vi "Adjust 1D Array to want Size.vi"(10 "y":i32=100, 11 "1D Input":dbl[](array[numeric])) -> (3 "1D Output":dbl[](array[numeric]))   [LabVIEW 2021]
doc: "向HMI写数组时，先在HMI里面配置X和Y的数组大小，OPC里面限制float大小为127，实际使用100.\n当写入的数组不等于100时，HMI上面不显示波形。\n故要调整输入数组的大小。多的去掉，小的补充。\n2015-05-26 09:55:54\n蒋松\njiangsong@outlook.com"
panel:
  out "Waveform Graph":dbl[](graph)
  out "size(s)":i32
  in  "Numeric":i32
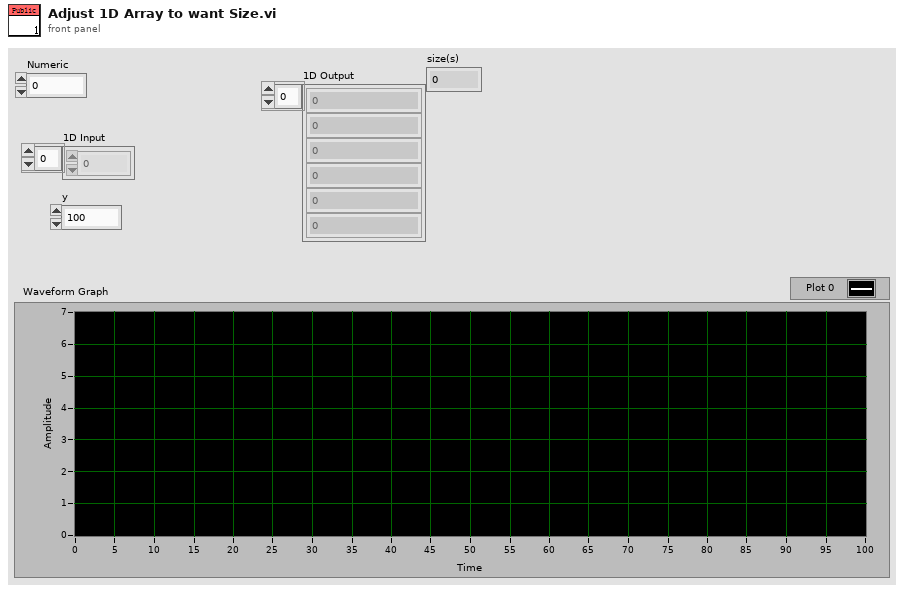
[diagram p1: front panel]
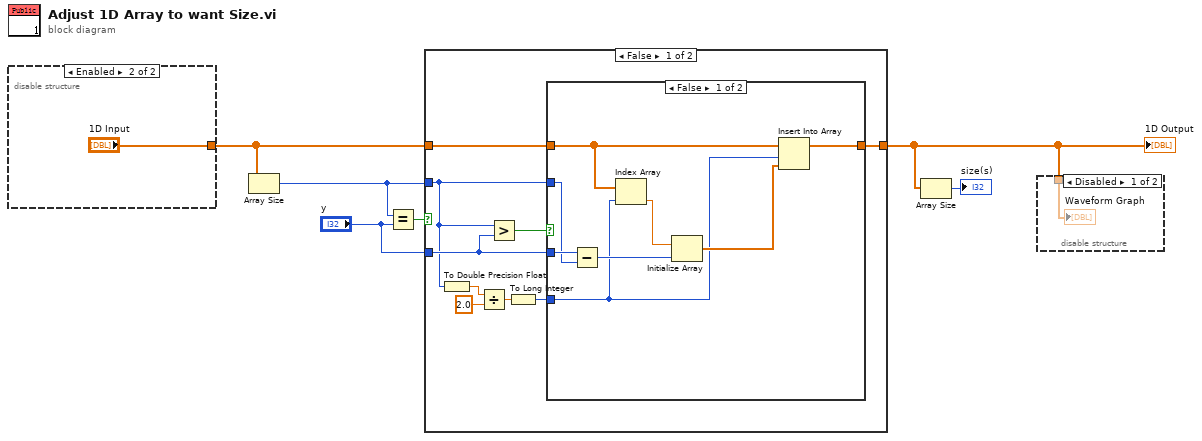
[diagram p0: block diagram]
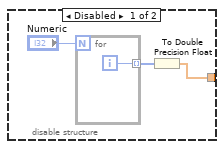
[diagram p3: hidden frame]
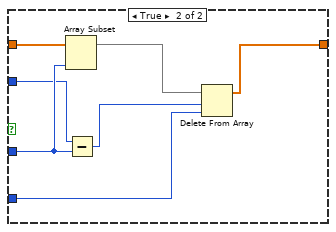
[diagram p4: hidden frame]
diagram:
  n1 = disable-structure shown="Enabled" {
    disable-tunnel: [w7 "1D Input"] -> w3
    frame Disabled {
      n2 = for {
        N: "Numeric" -> [_]
        tunnel: [w10] -> w8 mode=indexing
        i -> [w10]
      }
      n3 = To Double Precision Float(number=w8) -> (double precision float=w7:dbl[])
    }
    frame Enabled {
    }
  }
  n4 = Array Size(array=w3) -> (size(s)=w5:i32)
  n5 = Equal?(x=w5, y="y") -> (x = y?=w6:bool)
  n6 = case shown="False" w6 {
    tunnel: [w18 w36] -> w1
    tunnel: w3 -> [w19 w36]
    tunnel: w5 -> [w13 _]
    tunnel: "y" -> [w17 _]
    frame False {
      n7 = To Double Precision Float(number=w13) -> (double precision float=w15:dbl)
      n8 = Divide(x=w15, y=2.0) -> (x/y=w16:dbl)
      n9 = Greater?(x=w13, y=w17) -> (0:w20:bool)
      n10 = To Long Integer(number=w16) -> (32bit integer=w12:i32)
      n11 = case shown="False" w20 {
        tunnel: w19 -> [w25 w35]
        tunnel: [w23 w30] -> w18
        tunnel: w17 -> [w28 w34]
        tunnel: w13 -> [w22 w32]
        tunnel: w12 -> [w21 w29]
        frame False {
          n12 = Subtract(x=w28, y=w22) -> (x-y=w26:i32)
          n13 = Index Array(array=w25, index=w21) -> (element=w27:dbl)
          n14 = Initialize Array(w27, w26) -> (w24:dbl[])
          n15 = Insert Into Array(array=w25, index=w21, new element=w24) -> (w23:dbl[])
        }
        frame True {
          n16 = Array Subset(array=w35, length=w34) -> (w31:dbl[])  [unwired: 1 in]
          n17 = Subtract(x=w32, y=w34) -> (x-y=w33:i32)
          n18 = Delete From Array(array=w31, length=w33, index=w29) -> (array with subset deleted=w30:dbl[])  [unwired: 1 out]
        }
      }
    }
    frame True {
    }
  }
  "1D Output" <- w1
  n19 = Array Size(array=w1) -> (size(s)=→"size(s)":i32)
  n20 = disable-structure shown="Disabled" {
    disable-tunnel: w1 -> [w37 _]
    frame Disabled {
      "Waveform Graph" <- w37
    }
    frame Enabled {
    }
  }
